vi "test_Set and Get 9227.vi"(8 "error in (no error)":errorcluster, 11 "TestCase in":refnum<class "Scan Engine Scripting API Custom Device Unit Tests.lvclass">) -> (0 "error out":errorcluster, 3 "TestCase out":refnum<class "Scan Engine Scripting API Custom Device Unit Tests.lvclass">)   [LabVIEW 2017, in "Scan Engine Scripting API Custom Device Unit Tests.lvclass"]
uses:
  Scan Engine Scripting API Custom Device Unit Tests.lvclass
  Scan Engine Scripting API Custom Device Unit Tests.lvclass/Scan Engine Scripting API Custom Device Unit Tests.ctl
  Scripting/Modules/NI 9227/NI 9227.lvclass
  C:/dev/niveristand-scan-engine-ethercat-custom-device/Custom Device Source/Scripting/Modules/Module/Module.lvclass
  <vilib>/addons/_JKI Toolkits/VI Tester/TestCase.llb/TestCase.lvclass
  Scripting/Scan Engine Scripting.lvlib
  C:/Program Files (x86)/National Instruments/LabVIEW 2017/vi.lib/addons/_JKI Toolkits/VI Tester/TestCase.llb/TestCase.lvclass
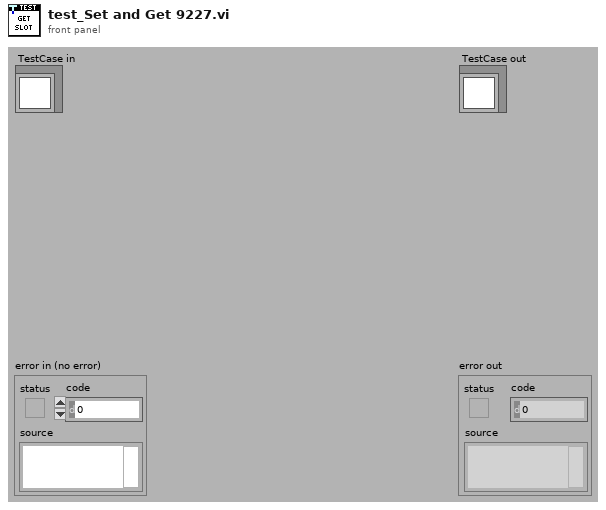
[diagram p1: front panel]
types:
  T1 = typedef "Custom Device API.lvlib/Custom Device Item Ref.ctl" = u64
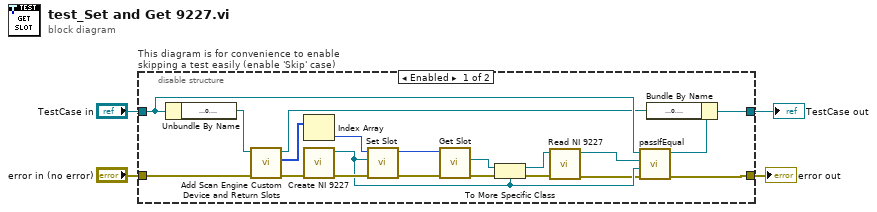
[diagram p0: block diagram]
diagram:
  n1 = disable-structure "This diagram is for convenience to enable skipping a test easily (enable 'Skip' case)" shown="Enabled" {
    disable-tunnel: "TestCase in" -> [w16 w28]
    disable-tunnel: [w20 w26] -> w1
    disable-tunnel: [w11 w27] -> w3
    disable-tunnel: "error in (no error)" -> [w24 w25]
    frame Enabled {
      n2 = Unbundle By Name(w16) -> ("target ref"=w23:refnum<k24>)
      n3 = call "Add Scan Engine Custom Device and Return Slots.vi"("error in"=w24, "target ref in"=w23) -> ("error out"=w14:errorcluster, "slot refs"=w22:T1[], "target ref out"=w15:refnum<k24>)  [unwired: 7 in]
      n4 = Index Array(array=w22) -> (element=w21:T1)  [unwired: 1 in]
      n5 = call "Create NI 9227.vi"("error in"=w14) -> ("error out"=w13:errorcluster, "NI 9227 out"=w8:refnum<class "NI 9227.lvclass">)  [unwired: 9 in]
      n6 = call "Set Slot.vi"("error in"=w13, "module"=w8, "slot ref in"=w21) -> ("error out"=w19:errorcluster, "slot ref out"=w5:T1)  [unwired: 7 in]
      n7 = call "Get Slot.vi"("error in"=w19, "slot ref in"=w5) -> ("error out"=w18:errorcluster, "module"=w17:refnum<class "Module.lvclass">)  [unwired: 6 in, 2 out]
      n8 = To More Specific Class(target class=w8, reference=w17, error in=w18) -> (specific class reference=w10:refnum<class "NI 9227.lvclass">, error out=w12:errorcluster)
      n9 = call "Read NI 9227.vi"("error in"=w12, "NI 9227 in"=w10) -> ("error out"=w7:errorcluster, "NI 9227 out"=w9:refnum<class "NI 9227.lvclass">)  [unwired: 7 in, 1 out]
      n10 = call-dynamic "passIfEqual.vi"("error in (no error)"=w7, "y"=w8, "x"=w9, "TestCase in"=w16) -> ("error out"=w11:errorcluster, "TestCase out"=w6:refnum<class "Scan Engine Scripting API Custom Device Unit Tests.lvclass">)  [unwired: 6 in]
      n11 = Bundle By Name(cluster=w6, "target ref"=w15) -> (w20:refnum<class "Scan Engine Scripting API Custom Device Unit Tests.lvclass">)
    }
    frame Disabled {
      # "skip test result while test is under development"
      n12 = call <vilib>:"skip.vi"("error in (no error)"=w25, "TestCase in"=w28) -> ("error out"=w27:errorcluster, "TestCase out"=w26:refnum<class "Scan Engine Scripting API Custom Device Unit Tests.lvclass">)  [unwired: 8 in]
    }
  }
  "error out" <- w3
  "TestCase out" <- w1
